vi "Test Status Update Bug.vi"(8 "error in (no error)":errorcluster) -> (0 "error out":errorcluster)   [LabVIEW 2013]
uses:
  classes/Test Suite/Test Suite.lvclass
  classes/Test Suite/Define Test Suite (SimpleText Report).vi
panel:
  out "Test Report File Contents":string
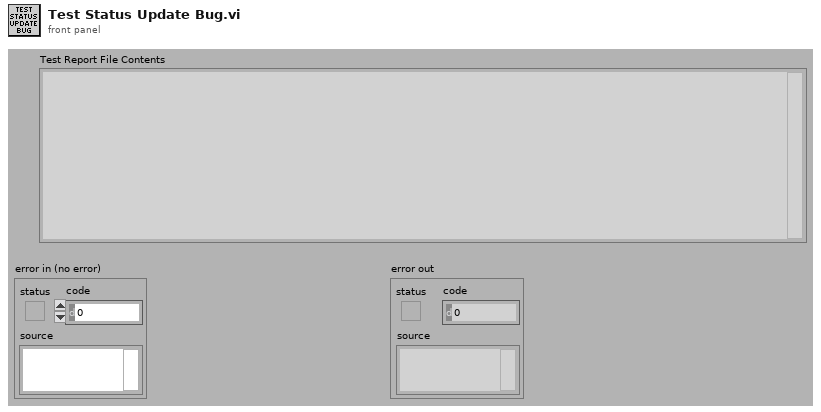
[diagram p1: front panel]
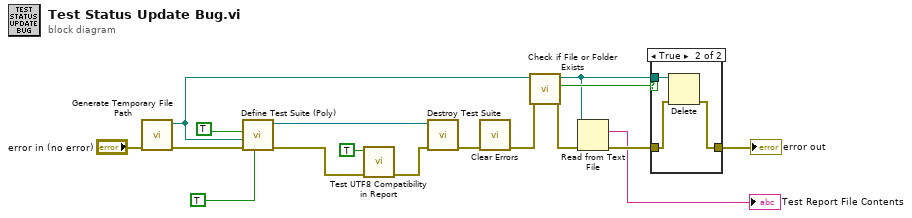
[diagram p0: block diagram]
diagram:
  n1 = call <vilib>:"Generate Temporary File Path.vi"("error in (no error)"="error in (no error)") -> ("error out"=w8:errorcluster, "Unique Temporary File Path"=w7:path)  [unwired: 9 in]
  n2 = call-poly "Define Test Suite (Poly).vi"("Verbose (F)"=TRUE, "error in (no error)"=w8, "Report Path"=w7, "Interactive"=TRUE) -> ("error out"=w6:errorcluster, "Test Suite"=w9:refnum<class "Test Suite.lvclass">)  [unwired: 5 in, 1 out]
  n3 = call "Test UTF8 Compatibility in Report.vi"("error in (no error)"=w6, "Force FAIL?"=TRUE) -> ("error out"=w1:errorcluster)  [unwired: 9 in]
  n4 = call-dynamic "Destroy Test Suite.vi"("error in (no error)"=w1, "Test Suite in"=w9) -> ("error out"=w4:errorcluster)  [unwired: 8 in, 1 out]
  n5 = call <vilib>:"Clear Errors.vi"("error in (no error)"=w4) -> ("error out"=w3:errorcluster)  [unwired: 6 in]
  n6 = call <vilib>:"Check if File or Folder Exists.vi"("error in (no error)"=w3, "path"=w7) -> ("error out"=w14:errorcluster, "file or folder exists?"=w16:bool, "dup path"=w11:path)  [unwired: 7 in]
  n7 = Read from Text File(file (use dialog)=w11, error in=w14) -> (text=→"Test Report File Contents":string, error out=w13:errorcluster)  [unwired: 2 in, 2 out]
  n8 = case shown="True" w16 {
    tunnel: w11 -> [_ w21]
    tunnel: w13 -> [w18 w20]
    tunnel: [w18 w19] -> w15
    frame False {
    }
    frame True {
      n9 = Delete(path (use dialog)=w21, error in=w20) -> (error out=w19:errorcluster)  [unwired: 3 in, 2 out]
    }
  }
  "error out" <- w15
